vi "Main_Code.vi"() -> ()   [LabVIEW 2020]
uses:
  <vilib>/httpClient/POSTBuffer.vi
  <vilib>/httpClient/LabVIEWHTTPClient.lvlib
panel:
  in  "Minutos Inseridos\n(Portal)":dbl=1.0 format="%#_13g"
  in  "Tempo entre testes\n(Minutos)":dbl=1.0 format="%#_13g"
  out "comparador":string
  out "limiter":string
  in  "Start/Stop":bool
  out "A hora final inserida é compatível com a recebida?":bool
  out "hora_final":string
  out "A hora inicial inserida é compatível com a recebida?":bool
  out "hora_inicial":string
  out "A data inserida é compatível com a recebida?":bool
  out "data":string
  out "A conexão foi concluída?":bool
  out "body":string
  out "headers":string
  in  "ProjectID":string
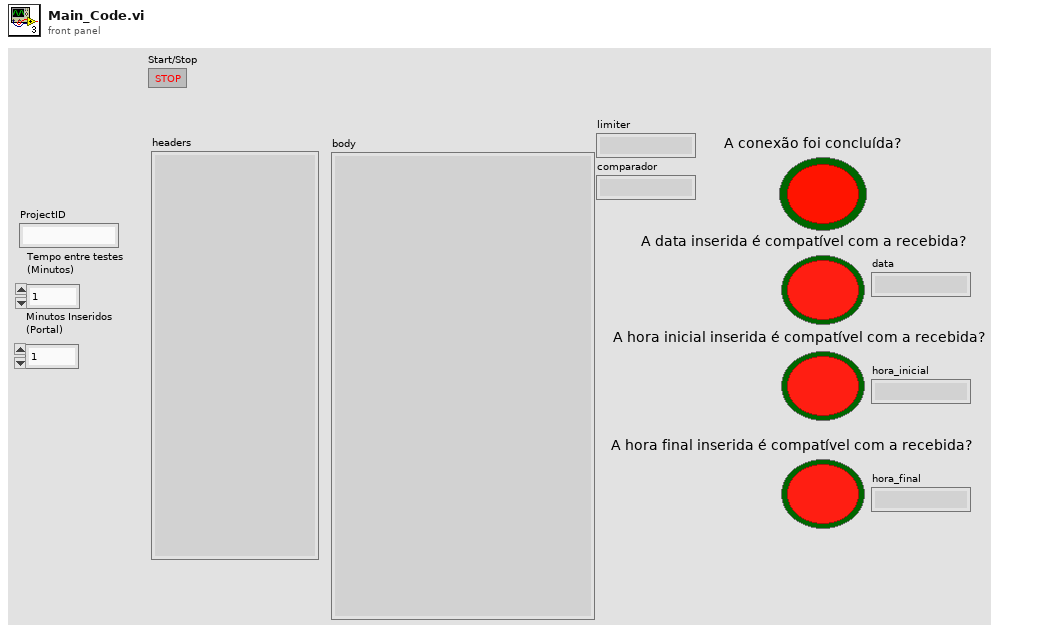
[diagram p1: front panel]
types:
  T1 = typedef "LabVIEWHTTPClient.lvlib/ClientHandle.ctl" = refnum<k1>
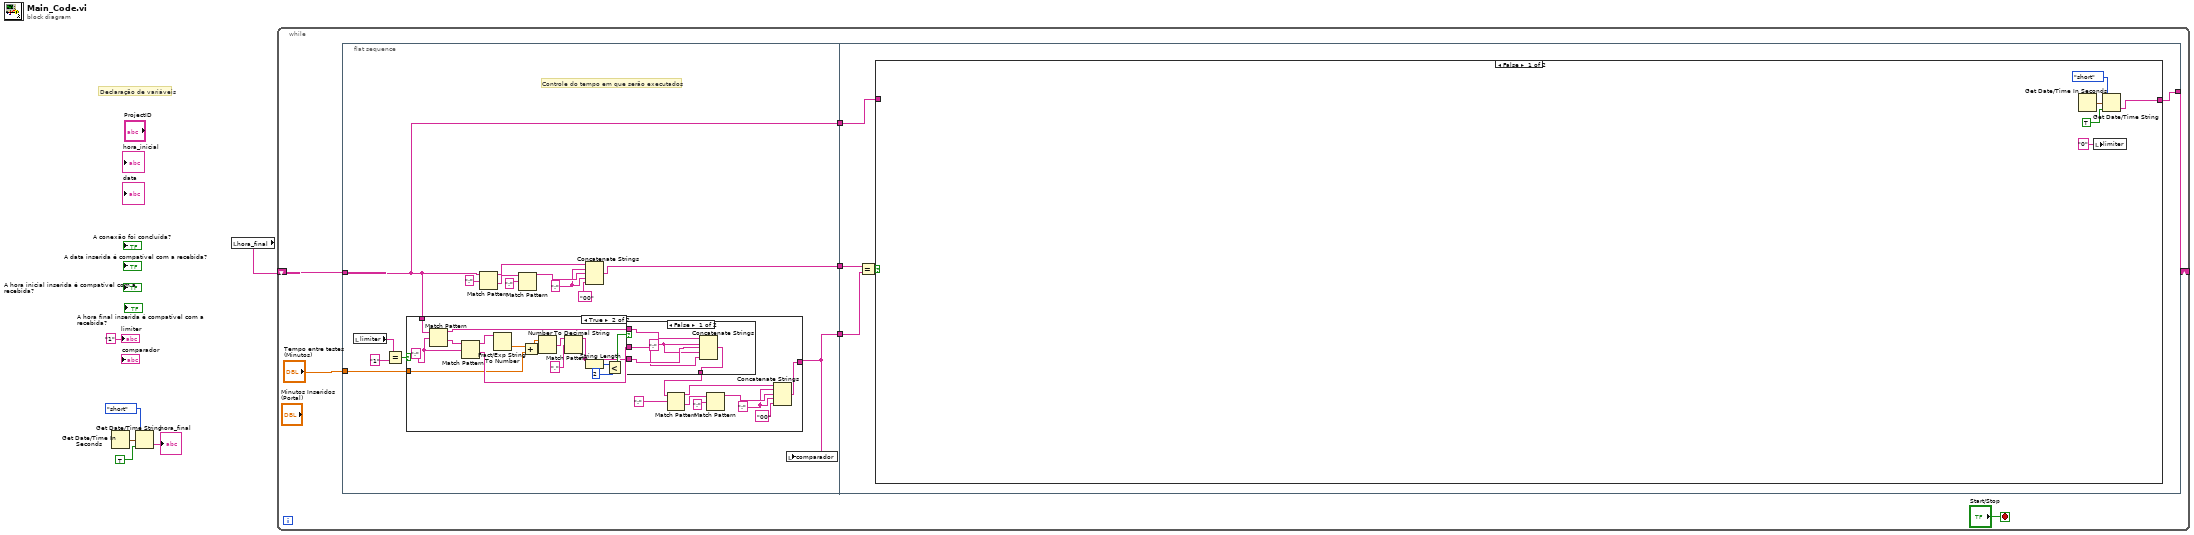
[diagram p0: block diagram]
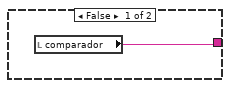
[diagram p2: hidden frame]
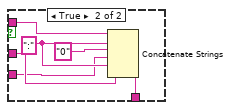
[diagram p3: hidden frame]
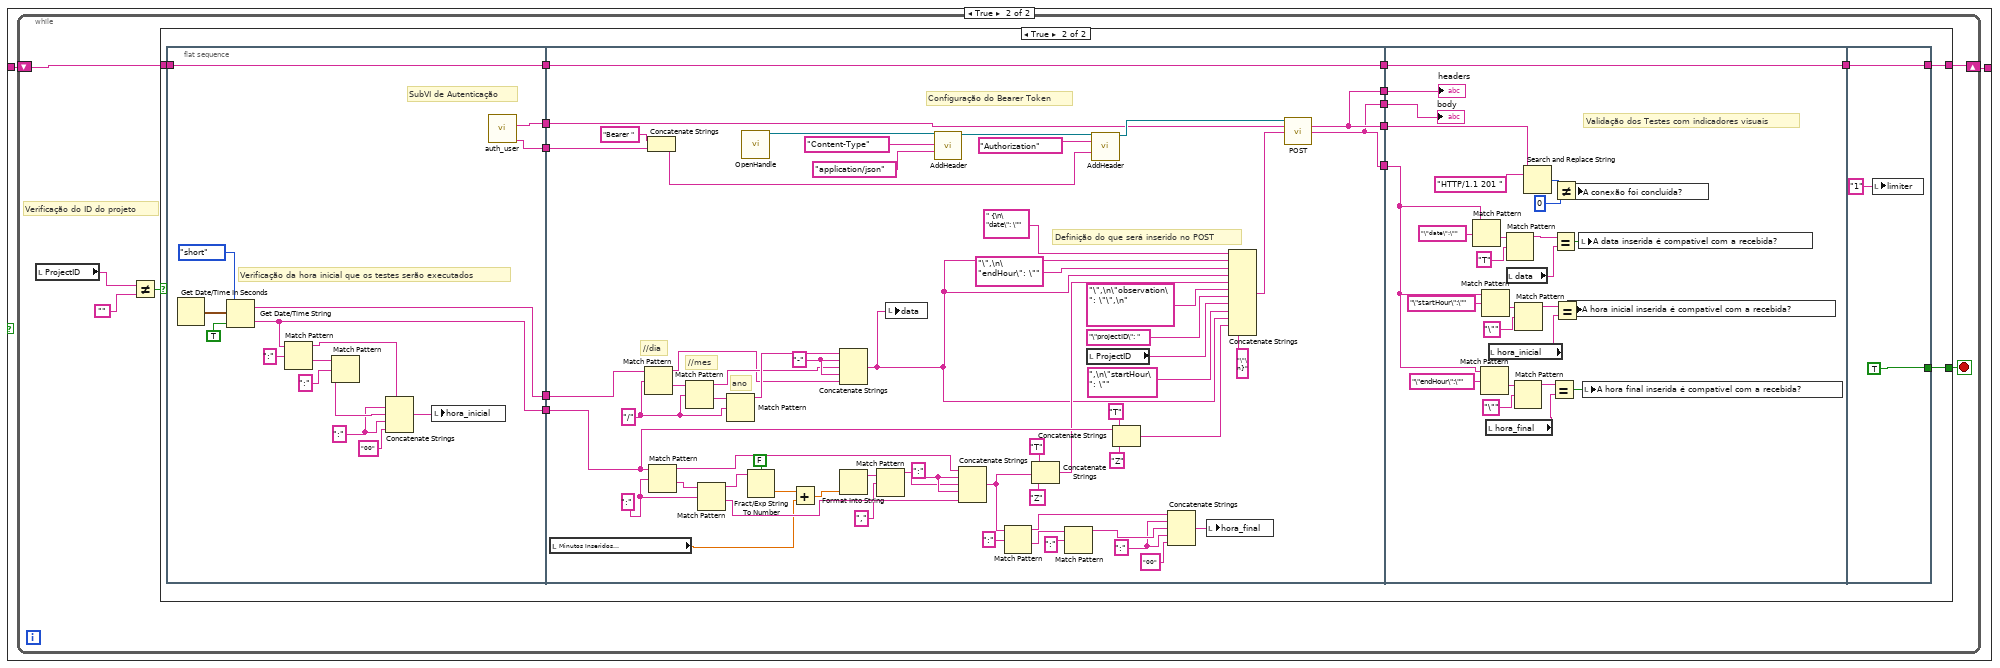
[diagram p4: hidden frame]
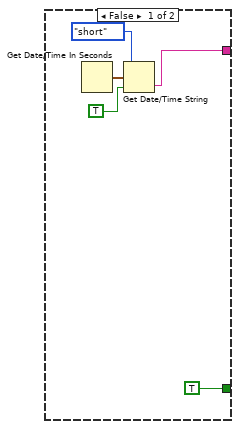
[diagram p5: hidden frame]
diagram:
  # "Declaração de variáveis"
  n1 = Get Date/Time In Seconds() -> (seconds since 1Jan1904=w6:timestamp)
  n2 = Get Date/Time String(date format (0)=enum16{"short", "long", "abbreviated"}."short", seconds (now)=w6, want seconds? (F)=TRUE) -> (time string=→"hora_final":string)  [unwired: 1 out]
  n3 = local read "hora_final"() -> (w2:string)
  n4 = while {
    shift-right: [w9] -> _
    shift-left: w2 -> [w13]
    stop <- "Start/Stop" stop-if-true
    n5 = flat-sequence {
      tunnel: w13 -> [w19]
      tunnel: [w20] -> w12
      tunnel: [w15] -> w11
      tunnel: [w19] -> w10
      tunnel: "Tempo entre testes\n(Minutos)" -> [w14]
      tunnel: w12 -> [w68]
      tunnel: w11 -> [w64]
      tunnel: w10 -> [w67]
      tunnel: [w66] -> w9
      frame #0 {
        w23 = ":" ("string")
        # "Controle do tempo em que serão executados"
        n6 = local read "limiter"() -> (w17:string)
        n7 = Equal?(x=w17, y="1") -> (x = y?=w18:bool)
        n8 = case shown="True" w18 {
          tunnel: [w28 w38] -> w15
          tunnel: w19 -> [_ w37]
          tunnel: w14 -> [_ w29]
          frame False {
            n9 = local read "comparador"() -> (w28:string)
          }
          frame True {
            w41 = ":" ("string")
            w51 = ":" ("regular expression")
            n10 = Match Pattern(string=w37, regular expression=w51) -> (before substring=w47:string, after substring=w52:string)  [unwired: 1 in, 2 out]
            n11 = Match Pattern(string=w52, regular expression=w51) -> (before substring=w48:string, after substring=w46:string)  [unwired: 1 in, 2 out]
            n12 = Fract/Exp String To Number(string=w48) -> (number=w50:dbl)  [unwired: 3 in, 1 out]
            n13 = Add(x=w50, y=w29) -> (x+y=w36:dbl)
            n14 = Number To Decimal String(number=w36) -> (decimal integer string=w35:string)  [unwired: 1 in]
            n15 = Match Pattern(string=w35, regular expression=",") -> (before substring=w30:string)  [unwired: 1 in, 3 out]
            n16 = String Length(string=w30) -> (length=w34:i32)
            n17 = Less?(x=w34, y=2) -> (x < y?=w32:bool)
            n18 = case shown="False" w32 {
              tunnel: w47 -> [w57 w63]
              tunnel: w46 -> [w53 w60]
              tunnel: [w56 w62] -> w31
              tunnel: w30 -> [w55 w58]
              frame False {
                w54 = ":" ("string")
                n19 = Concatenate Strings(w57, w54, w55, w54, w53) -> (w56:string)
              }
              frame True {
                w61 = ":" ("string")
                n20 = Concatenate Strings(w63, w61, "0" ("string"), w58, w61, w60) -> (w62:string)
              }
            }
            n21 = Match Pattern(string=w31, regular expression=":") -> (before substring=w39:string, after substring=w43:string)  [unwired: 1 in, 2 out]
            n22 = Match Pattern(string=w43, regular expression=":") -> (before substring=w42:string)  [unwired: 1 in, 3 out]
            n23 = Concatenate Strings(w39, w41, w42, w41, "00" ("string")) -> (w38:string)
          }
        }
        n24 = Match Pattern(string=w19, regular expression=":") -> (before substring=w21:string, after substring=w25:string)  [unwired: 1 in, 2 out]
        n25 = Match Pattern(string=w25, regular expression=":") -> (before substring=w24:string)  [unwired: 1 in, 3 out]
        n26 = Concatenate Strings(w21, w23, w24, w23, "00" ("string")) -> (w20:string)
        n27 = local write "comparador"(w15) -> ()
      }
      frame #1 {
        n28 = Equal?(x=w68, y=w64) -> (x = y?=w65:bool)
        n29 = case shown="False" w65 {
          tunnel: w67 -> [_ w75]
          tunnel: [w69 w74] -> w66
          frame False {
            n30 = Get Date/Time In Seconds() -> (seconds since 1Jan1904=w72:timestamp)
            n31 = local write "limiter"("0" ("limiter")) -> ()
            n32 = Get Date/Time String(date format (0)=enum16{"short", "long", "abbreviated"}."short", seconds (now)=w72, want seconds? (F)=TRUE) -> (time string=w69:string)  [unwired: 1 out]
          }
          frame True {
            n33 = while {
              shift-right: [w76] -> w74
              shift-left: w75 -> [w77]
              stop <- w78 stop-if-true
              # "Verificação do ID do projeto"
              n34 = local read "ProjectID"() -> (w80:string)
              n35 = Not Equal?(x=w80, y="") -> (x != y?=w81:bool)
              n36 = case shown="True" w81 {
                tunnel: [TRUE w92] -> w78
                tunnel: w77 -> [_ w91]
                tunnel: [w82 w87] -> w76
                frame False {
                  n37 = Get Date/Time In Seconds() -> (seconds since 1Jan1904=w85:timestamp)
                  n38 = Get Date/Time String(date format (0)=enum16{"short", "long", "abbreviated"}."short", seconds (now)=w85, want seconds? (F)=TRUE) -> (time string=w82:string)  [unwired: 1 out]
                }
                frame True {
                  n39 = flat-sequence {
                    tunnel: [w116] -> w100
                    tunnel: [w115] -> w99
                    tunnel: [w111] -> w98
                    tunnel: [w105] -> w97
                    tunnel: w91 -> [w101]
                    tunnel: [w101] -> w90
                    tunnel: w100 -> [w166]
                    tunnel: w99 -> [w168]
                    tunnel: w98 -> [w162]
                    tunnel: w97 -> [w139]
                    tunnel: [w130] -> w96
                    tunnel: [w129] -> w95
                    tunnel: [w130] -> w94
                    tunnel: [w129] -> w93
                    tunnel: w90 -> [w118]
                    tunnel: [w118] -> w88
                    tunnel: w96 -> [w202]
                    tunnel: w95 -> [w177]
                    tunnel: w94 -> [w179]
                    tunnel: w93 -> [w178]
                    tunnel: [w176] -> w89
                    tunnel: w88 -> [w176]
                    tunnel: [TRUE] -> w92
                    tunnel: [w204] -> w87
                    tunnel: w89 -> [w204]
                    frame #0 {
                      w107 = ":" ("string")
                      # "SubVI de Autenticação"
                      # "Verificação da hora inicial que os testes serão executados"
                      n40 = Get Date/Time In Seconds() -> (seconds since 1Jan1904=w113:timestamp)
                      n41 = Get Date/Time String(date format (0)=enum16{"short", "long", "abbreviated"}."short", seconds (now)=w113, want seconds? (F)=TRUE) -> (date string=w111:string, time string=w105:string)
                      n42 = Match Pattern(string=w105, regular expression=":") -> (before substring=w102:string, after substring=w104:string)  [unwired: 1 in, 2 out]
                      n43 = Match Pattern(string=w104, regular expression=":") -> (before substring=w108:string)  [unwired: 1 in, 3 out]
                      n44 = Concatenate Strings(w102, w107, w108, w107, "00" ("string")) -> (w103:string)
                      n45 = local write "hora_inicial"(w103) -> ()
                      n46 = call "auth_user.vi"() -> ("tokenReceiver"=w115:string, "urlbodyPost"=w116:string)  [unwired: 9 in, 1 out]
                    }
                    frame #1 {
                      w122 = ":" ("string")
                      w148 = "-" ("string")
                      w151 = ":"
                      w154 = ":" ("regular expression")
                      w158 = "/" ("regular expression")
                      # "Configuração do Bearer Token"
                      # "Definição do que será inserido no POST"
                      # "ano"
                      # "//mes"
                      # "//dia"
                      n47 = local read "Minutos Inseridos\n(Portal)"() -> (w117:dbl)
                      n48 = Match Pattern(string=w162, regular expression=w158) -> (before substring=w146:string, after substring=w161:string)  [unwired: 1 in, 2 out]
                      n49 = Concatenate Strings("Bearer ", w168) -> (w169:string)
                      n50 = Match Pattern(string=w139, regular expression=w154) -> (before substring=w155:string, after substring=w159:string)  [unwired: 1 in, 2 out]
                      n51 = Match Pattern(string=w161, regular expression=w158) -> (before substring=w147:string, after substring=w160:string)  [unwired: 1 in, 2 out]
                      n52 = Match Pattern(string=w159, regular expression=w154) -> (before substring=w157:string, after substring=w150:string)  [unwired: 1 in, 2 out]
                      n53 = Match Pattern(string=w160, regular expression=w158) -> (before substring=w149:string)  [unwired: 1 in, 3 out]
                      n54 = call <vilib>:"OpenHandle.vi"() -> ("client handle out"=w175:T1)  [unwired: 14 in, 1 out]
                      n55 = Fract/Exp String To Number(use system decimal point (T)=FALSE, string=w157) -> (number=w153:dbl)  [unwired: 2 in, 1 out]
                      n56 = Add(x=w153, y=w117) -> (x+y=w152:dbl)
                      n57 = Concatenate Strings(w149, w148, w147, w148, w146) -> (w128:string)
                      n58 = Format Into String(w152) -> (resulting string=w136:string)  [unwired: 3 in, 1 out]
                      n59 = Match Pattern(string=w136, regular expression=",") -> (before substring=w134:string)  [unwired: 1 in, 3 out]
                      n60 = local write "data"(w128) -> ()
                      n61 = call <vilib>:"AddHeader.vi"("client handle"=w175, "header"="Content-Type", "value"="application/json") -> ("client handle out"=w172:T1)  [unwired: 11 in, 1 out]
                      n62 = Concatenate Strings(w155, w151, w134, w151, w150) -> (w127:string)
                      n63 = Match Pattern(string=w127, regular expression=":") -> (before substring=w119:string, after substring=w124:string)  [unwired: 1 in, 2 out]
                      n64 = Concatenate Strings("T" ("string"), w127, "Z" ("string")) -> (w133:string)
                      n65 = Match Pattern(string=w124, regular expression=":") -> (before substring=w123:string)  [unwired: 1 in, 3 out]
                      n66 = local read "ProjectID"() -> (w143:string)
                      n67 = call <vilib>:"AddHeader.vi"("client handle"=w172, "header"="Authorization", "value"=w169) -> ("client handle out"=w167:T1)  [unwired: 11 in, 1 out]
                      n68 = Concatenate Strings("T" ("string"), w139, "Z" ("string")) -> (w138:string)
                      n69 = Concatenate Strings(w119, w122, w123, w122, "00" ("string")) -> (w120:string)
                      n70 = local write "hora_final"(w120) -> ()
                      n71 = Concatenate Strings(" {\n\"date\": \"", w128, "\",\n\"endHour\": \"" ("string"), w128, w133, "\",\n\"observation\": \"\",\n" ("string"), "\"projectID\": " ("string"), w143, ",\n\"startHour\": \"" ("string"), w128, w138, "\"\n}" ("string")) -> (w165:string)
                      n72 = call-poly <vilib>:"POST.vi"("client handle"=w167, "url"=w166, "buffer"=w165) -> ("headers"=w130:string, "body"=w129:string)  [unwired: 9 in, 2 out]
                    }
                    frame #2 {
                      # "Validação dos Testes com indicadores visuais"
                      n73 = Match Pattern(string=w177, regular expression="\"date\":\"") -> (after substring=w196:string)  [unwired: 1 in, 3 out]
                      n74 = Match Pattern(string=w177, regular expression="\"endHour\":\"") -> (after substring=w184:string)  [unwired: 1 in, 3 out]
                      n75 = Match Pattern(string=w177, regular expression="\"startHour\":\"") -> (after substring=w190:string)  [unwired: 1 in, 3 out]
                      n76 = local read "hora_final"() -> (w181:string)
                      n77 = local read "hora_inicial"() -> (w187:string)
                      n78 = Match Pattern(string=w196, regular expression="T") -> (before substring=w194:string)  [unwired: 1 in, 3 out]
                      n79 = local read "data"() -> (w193:string)
                      n80 = Match Pattern(string=w184, regular expression="\"") -> (before substring=w182:string)  [unwired: 1 in, 3 out]
                      n81 = Match Pattern(string=w190, regular expression="\"") -> (before substring=w188:string)  [unwired: 1 in, 3 out]
                      n82 = Search and Replace String(input string=w202, search string="HTTP/1.1 201 ") -> (number of replacements=w200:i32)  [unwired: 6 in, 3 out]
                      n83 = Equal?(x=w182, y=w181) -> (x = y?=w180:bool)
                      n84 = Equal?(x=w194, y=w193) -> (x = y?=w192:bool)
                      n85 = Not Equal?(x=w200, y=0) -> (x != y?=w198:bool)
                      n86 = Equal?(x=w188, y=w187) -> (x = y?=w186:bool)
                      n87 = local write "A hora inicial inserida é compatível com a recebida?"(w186) -> ()
                      n88 = local write "A conexão foi concluída?"(w198) -> ()
                      n89 = local write "A data inserida é compatível com a recebida?"(w192) -> ()
                      n90 = local write "A hora final inserida é compatível com a recebida?"(w180) -> ()
                      "headers" <- w179
                      "body" <- w178
                    }
                    frame #3 {
                      n91 = local write "limiter"("1" ("limiter")) -> ()
                    }
                  }
                }
              }
            }
          }
        }
      }
    }
  }
  "limiter" <- "1" ("limiter")
